vi "Prova.vi"   [LabVIEW 2016]
uses:
  <userlib>/LVLibSVM/LibSVM Sparse/SubVIs/SVM Train NU_SVR.vi
  <userlib>/LVLibSVM/LibSVM Sparse/Wrapper API/svm_train.vi
types:
  T1 = typedef "svm_problem.ctl" = cluster{"y":dbl[], "x":cluster{T2[]}[]}
  T2 = typedef "svm_node.ctl" = cluster{"index":i32, "value":dbl}
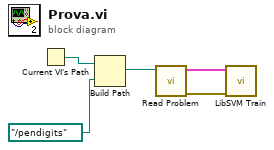
[diagram p0: block diagram]
diagram:
  n1 = Current VI's Path() -> (path=w2:path)
  n2 = Build Path(base path=w2, name or relative path=path "../pendigits") -> (appended path=w3:path)
  n3 = call <userlib>:"Read Problem.vi"("file path (use dialog)"=w3) -> ("error out"=w4:errorcluster, "svm_problem"=w5:T1)  [unwired: 9 in]
  n4 = call-poly <userlib>:"LibSVM Train.vi"("error in (no error)"=w4, "Problem"=w5) -> ()  [unwired: 8 in, 2 out]
